vi "GetIndexFromPathNumber.vi"(1 "Loop size":dbl, 2 "Input paths":path[](array[path])) -> (0 "Index output":i32[](array[numeric]))   [LabVIEW 2010]
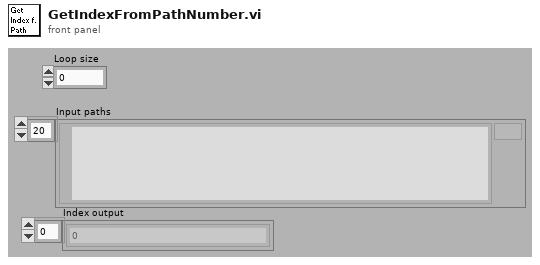
[diagram p1: front panel]
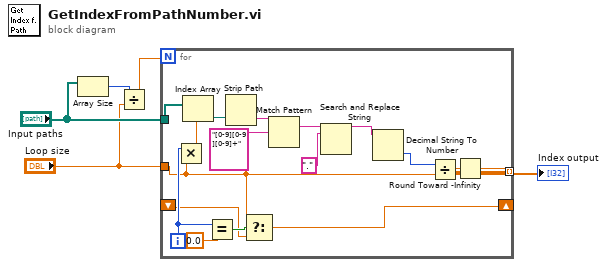
[diagram p0: block diagram]
diagram:
  n1 = Array Size(array="Input paths") -> (size(s)=w3:i32)
  n2 = Divide(x=w3, y="Loop size") -> (x/y=w1:dbl)
  n3 = for {
    N: w1 -> [_]
    tunnel: "Input paths" -> [w15]
    tunnel: "Loop size" -> [w9]
    tunnel: [w6] -> w5 mode=indexing
    shift-right: [w7] -> _
    shift-left: _ -> [w8]
    i -> [w12]
    n4 = Multiply(x=w12, y=w9) -> (x*y=w14:dbl)
    n5 = Index Array(array=w15, index=w14) -> (element=w13:path)
    n6 = Equal?(x=w12, y=0.0) -> (x = y?=w10:bool)
    n7 = Strip Path(path=w13) -> (name=w21:string)  [unwired: 1 out]
    n8 = Select(t=w9, s=w10, f=w8) -> (s? t:f=w7:dbl)
    n9 = Match Pattern(string=w21, regular expression="[0-9][0-9][0-9]+") -> (match substring=w20:string)  [unwired: 1 in, 3 out]
    n10 = Search and Replace String(input string=w20, search string=".") -> (result string=w18:string)  [unwired: 6 in, 3 out]
    n11 = Decimal String To Number(string=w18) -> (number=w17:i32)  [unwired: 2 in, 1 out]
    n12 = Divide(x=w17, y=w9) -> (x/y=w16:dbl)
    n13 = Round Toward -Infinity(1:w16) -> (0:w6:dbl)
  }
  "Index output" <- w5
